vi "Example Interrupt - Interrupt Callback.vi"(4 "Interrupt":refnum<user-event>, 5 "Event Data":T1, 6 "Control Ref":refnum<k24>, 7 "Event Common Data":T2) -> ()   [LabVIEW 2013]
uses:
  C:/tf/play/labview/Tinkerforge.dll
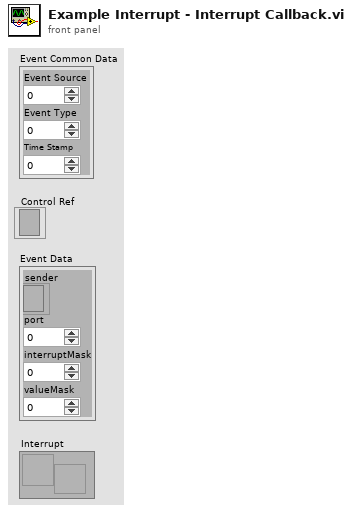
[diagram p1: front panel]
types:
  T1 = cluster{"sender":refnum<k24>, "port":u16, "interruptMask":u8, "valueMask":u8}
  T2 = cluster{"Event Source":i32, "Event Type":u32, "Time Stamp":u32}
  T3 = cluster{"port":u16, "interruptMask":u8, "valueMask":u8}
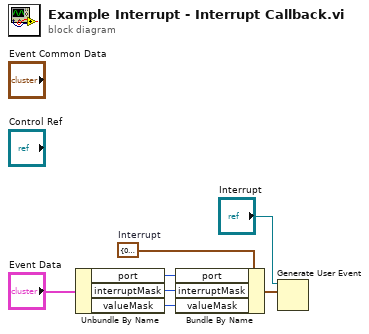
[diagram p0: block diagram]
diagram:
  w6 = T3 {"port"=0, "interruptMask"=0, "valueMask"=0}  # Interrupt
  n1 = Unbundle By Name("Event Data") -> ("port"=w5:u16, "interruptMask"=w4:u8, "valueMask"=w3:u8)
  n2 = Bundle By Name(cluster=w6, "port"=w5, "interruptMask"=w4, "valueMask"=w3) -> (w1:T3)
  n3 = Generate User Event(user event="Interrupt", event data cluster=w1) -> ()  [unwired: 2 in, 2 out]
